vi "Add I32Array to HashTable.vi"(8 "error in (no error)":errorcluster caption="错误输入（无错误）", 9 "Value":i32[](array[numeric]), 10 "Name":string[](array[string]), 11 "Contstant Base 输入":refnum<class "Tag Data.lvclass"> caption="DNL_LabVIEW Object in") -> (0 "error out":errorcluster caption="错误输出", 3 "Contstant Base 输出":refnum<class "Tag Data.lvclass"> caption="DNL_LabVIEW Object out")   [LabVIEW 2013, in "Tag Data.lvclass"]
uses:
  Tag Data.lvclass
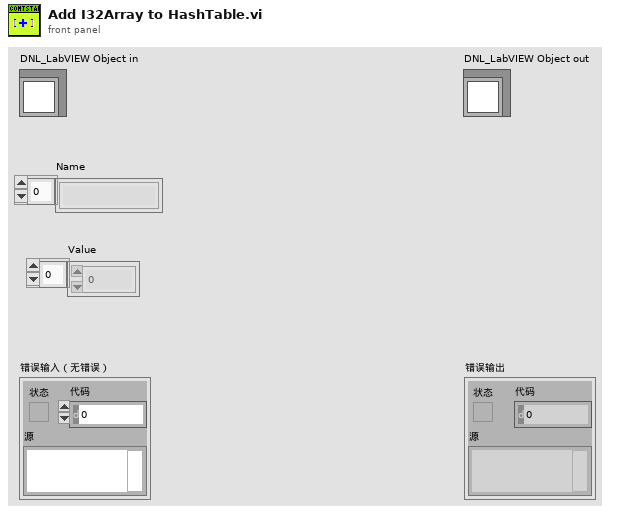
[diagram p1: front panel]
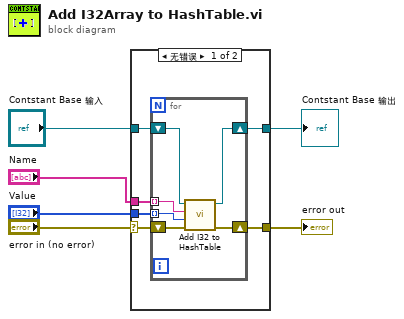
[diagram p0: block diagram]
diagram:
  n1 = case shown="无错误" "error in (no error)" {
    selector: "error in (no error)" -> [w10 w20]
    tunnel: [w9 w20] -> w5
    tunnel: [w7 w19] -> w3
    tunnel: "Contstant Base 输入" -> [w8 w19]
    tunnel: "Name" -> [w12 _]
    tunnel: "Value" -> [w11 _]
    frame No Error {
      n2 = for {
        tunnel: w12 -> [w18] mode=indexing
        tunnel: w11 -> [w17] mode=indexing
        shift-right: [w15] -> w9
        shift-left: w10 -> [w16]
        shift-right: [w13] -> w7
        shift-left: w8 -> [w14]
        n3 = call "Add I32 to HashTable.vi"("error in (no error)"=w16, "Value"=w17, "Name"=w18, "Contstant Base 输入"=w14) -> ("error out"=w15:errorcluster, "Contstant Base 输出"=w13:refnum<class "Tag Data.lvclass">)  [unwired: 6 in]
      }
    }
    frame Error {
    }
  }
  "error out" <- w5
  "Contstant Base 输出" <- w3
